vi "Medidor de som microfone.vi"() -> ()   [LabVIEW 2018]
uses:
  <vilib>/sound2/lvsound2.llb/Sampling Mode.ctl
  <vilib>/sound2/lvsound2.llb/Sound Data Format.ctl
  <vilib>/sound2/lvsound2.llb/Sound Input Read (DBL).vi
panel:
  out "Waveform Chart":waveform(dbl)[](graph)
  in  "stop":bool
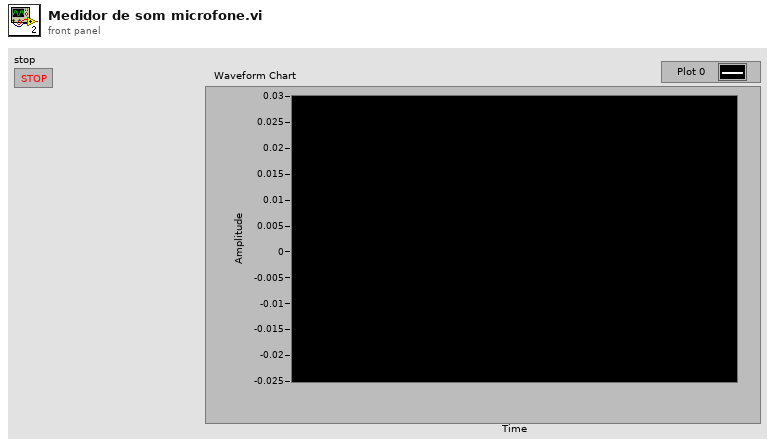
[diagram p1: front panel]
types:
  T1 = typedef "Sound Data Format.ctl" = cluster{"sample rate (S/s)":dbl, "number of channels":i32, "bits per sample":i32}
  T2 = typedef "Sampling Mode.ctl" = i32
  T3 = typedef "Sound Input Task ID.ctl" = u32
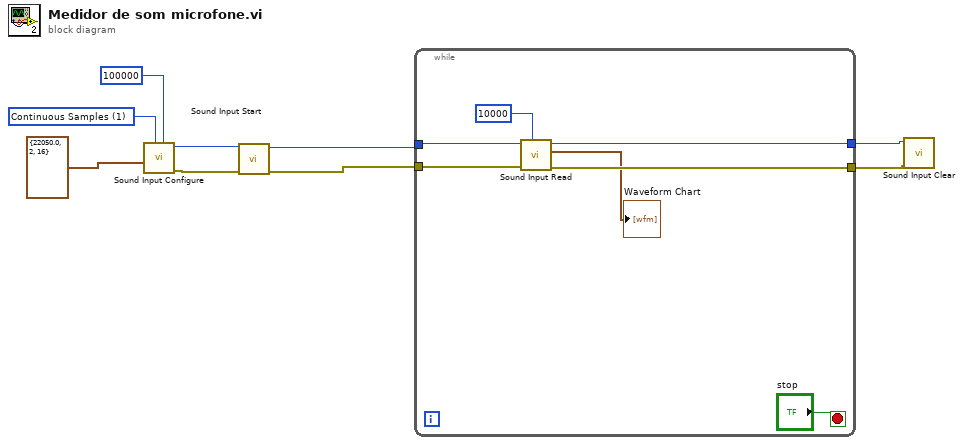
[diagram p0: block diagram]
diagram:
  w9 = T2 1 items=["Finite Samples", "Continuous Samples"] ("sample mode")
  n1 = call <vilib>:"Sound Input Configure.vi"("number of samples/ch"=100000, "sample mode"=w9, "sound format"=T1 {"sample rate (S/s)"=22050.0, "number of channels"=2, "bits per sample"=16}) -> ("error out"=w5:errorcluster, "task ID"=w6:T3)  [unwired: 7 in]
  n2 = call <vilib>:"Sound Input Start.vi"("error in (no error)"=w5, "task ID"=w6) -> ("error out"=w3:errorcluster, "task ID out"=w4:T3)  [unwired: 8 in]
  n3 = while {
    tunnel: w4 -> [w15]
    tunnel: w3 -> [w14]
    tunnel: [w11] -> w2
    tunnel: [w12] -> w1
    stop <- "stop" stop-if-true
    n4 = call-poly <vilib>:"Sound Input Read.vi"("number of samples/ch"=10000, "error in (no error)"=w14, "task ID"=w15) -> ("error out"=w12:errorcluster, "data"=→"Waveform Chart":waveform(dbl)[], "task ID out"=w11:T3)  [unwired: 6 in]
  }
  n5 = call <vilib>:"Sound Input Clear.vi"("error in (no error)"=w1, "task ID"=w2) -> ()  [unwired: 9 in, 1 out]
